vi "move folder contents up one hierarchy level.vi"(10 "error in":errorcluster, 11 "file":path) -> (2 "error out":errorcluster)   [LabVIEW 2014]
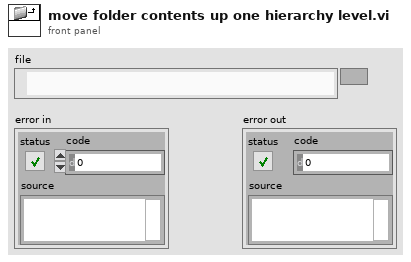
[diagram p1: front panel]
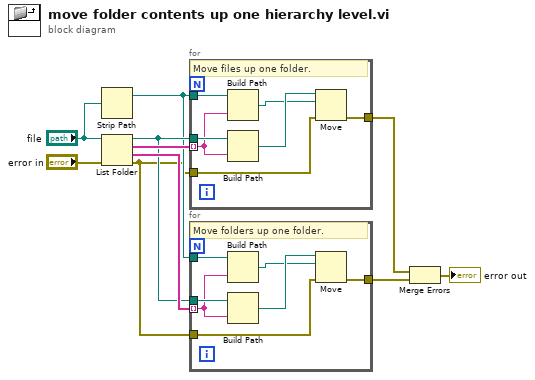
[diagram p0: block diagram]
diagram:
  n1 = Strip Path(path="file") -> (stripped path=w5:path)  [unwired: 1 out]
  n2 = List Folder(path="file", error in="error in") -> (path out=w6:path, filenames=w10:string[], folder names=w7:string[], error out=w4:errorcluster)  [unwired: 2 in]
  n3 = for {
    tunnel: w6 -> [w17]
    tunnel: w10 -> [w14] mode=indexing
    tunnel: w5 -> [w15]
    tunnel: w4 -> [w12]
    tunnel: [w11] -> w3
    # "Move files up one folder."
    n4 = Build Path(base path=w15, name or relative path=w14) -> (appended path=w13:path)
    n5 = Build Path(base path=w17, name or relative path=w14) -> (appended path=w16:path)
    n6 = Move(source path=w16, error in=w12, 10:w13) -> (error out=w11:errorcluster)  [unwired: 2 in, 2 out]
  }
  n7 = for {
    tunnel: w6 -> [w24]
    tunnel: w7 -> [w21] mode=indexing
    tunnel: w5 -> [w22]
    tunnel: w4 -> [w19]
    tunnel: [w18] -> w2
    # "Move folders up one folder."
    n8 = Build Path(base path=w22, name or relative path=w21) -> (appended path=w20:path)
    n9 = Build Path(base path=w24, name or relative path=w21) -> (appended path=w23:path)
    n10 = Move(source path=w23, error in=w19, 10:w20) -> (error out=w18:errorcluster)  [unwired: 2 in, 2 out]
  }
  n11 = Merge Errors(w3, w2) -> (→"error out":errorcluster)
